vi "FirewireGrab.vi"() -> ()   [LabVIEW 2009]
panel:
  in  "File Name":string
  out "Buoy Video":T1(plugin-control)
  in  "address":string="192.168.1.200"
  in  "?":string="To save a video file, enter file path location and hit enter.  To save another video change the file name and hit enter. \n"
  out "error out":errorcluster
  in  "stop":bool
  out "Filter Names":string[](array[string])
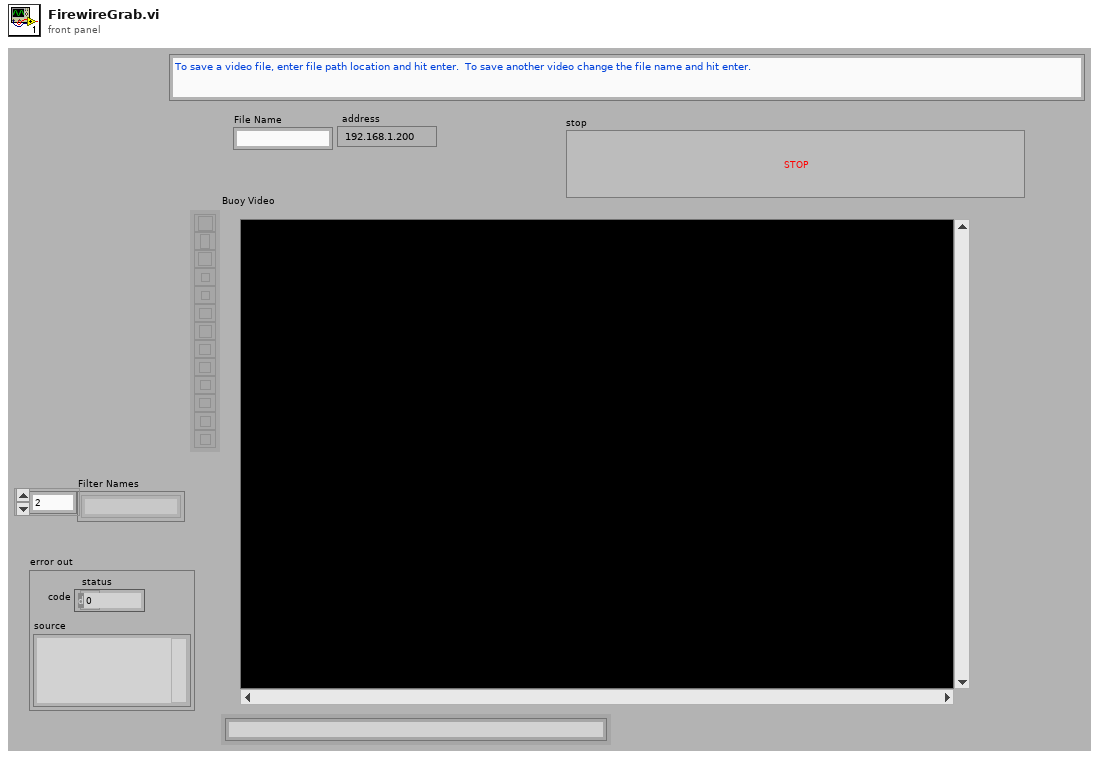
[diagram p1: front panel]
types:
  T1 = typedef "IMAQ Image.ctl" = refnum<image>
  T2 = enum16{"1280 x 1024 MJPG", "1280 x 960 MJPG", "1280 x 720 MJPG", "1280 x 480 MJPG", "640 x 480 MJPG", "320 x 240 MJPG", "160 x 120 MJPG"}
  T3 = typedef "AviRefnum.ctl" = refnum<k1>
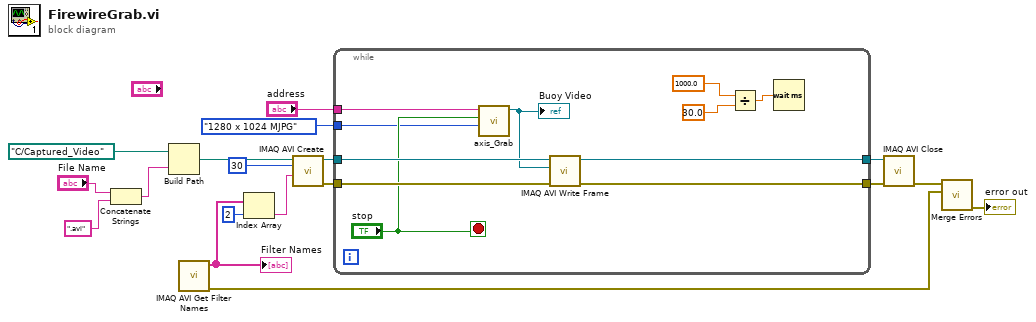
[diagram p0: block diagram]
diagram:
  n1 = Concatenate Strings("File Name", ".avi" ("string")) -> (w3:string)
  n2 = Build Path(base path=path "C:/Captured_Video" ("Save Location"), name or relative path=w3) -> (appended path=w4:path)
  n3 = call "IMAQ AVI Get Filter Names"() -> ("error out"=w9:errorcluster, "Filter Names"=w12:string[])  [unwired: 1 in, 9 out]
  "Filter Names" <- w12
  n4 = Index Array(array=w12, index=2) -> (element=w10:string)
  n5 = call "IMAQ AVI Create"("Compression Filter"=w10, "Frames Per Second"=u32 30, "AVI Path"=w4) -> ("error out"=w16:errorcluster, "Avi Refnum"=w17:T3)  [unwired: 4 in, 3 out]
  n6 = while {
    tunnel: w17 -> [w29]
    tunnel: w16 -> [w28]
    tunnel: [w27] -> w15
    tunnel: [w26] -> w14
    tunnel: "address" -> [w20]
    tunnel: T2."1280 x 1024 MJPG" ("Pixel Format") -> [w19]
    stop <- "stop" stop-if-true
    n7 = call "axis_Grab.vi"("Pixel Format"=w19, "stop"="stop", "address"=w20) -> ("Image"=w25:T1)  [unwired: 8 in]
    "Buoy Video" <- w25
    n8 = call "IMAQ AVI Write Frame"("error in (no error)"=w28, "Image"=w25, "Avi Refnum"=w29) -> ("error out"=w26:errorcluster, "Avi Refnum (duplicate)"=w27:T3)  [unwired: 1 in, 6 out]
    n9 = Divide(x=1000.0, y=30.0) -> (x/y=w23:dbl)
    n10 = Wait (ms)(milliseconds to wait=w23) -> ()  [unwired: 1 out]
  }
  n11 = call "IMAQ AVI Close"("error in (no error)"=w14, "Avi Refnum"=w15) -> ("error out"=w8:errorcluster)  [unwired: 9 out]
  n12 = call <vilib>:"Merge Errors.vi"("error in 2 (no error)"=w9, "error in 1 (no error)"=w8) -> ("error out"=→"error out":errorcluster)  [unwired: 2 in, 3 out]
